vi "Configure PuTTY Client.vi"   [LabVIEW 2020, in "NI_SSH.lvlib"]
doc: "Drops the code needed to pass additional configuration options to the OpenSSH client by wiring an PuTTY Client Constant into a Property Node."
uses:
  <vilib>/net/SSH/NI_SSH.lvlib
  <vilib>/net/SSH/Client/PuTTY/PuTTY Client.lvclass
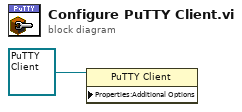
[diagram p0: block diagram]
diagram:
  n1 = property class="PuTTY Client" props=["Properties:Additional Options"](reference=refnum<class "PuTTY Client.lvclass"> refnum ("NI_SSH.lvlib:PuTTY Client")) -> ()  [unwired: 2 in, 2 out]
